vi "Validate Device ID Code.vi"(10 "Read Device ID code":T1, 11 "Device Conformity Level":T2=1 items=["None"=0, "Basic Stream"=1, "Regular Stream"=2, "Extended Stream"=3, "Basic Stream/Individual"=129, "Regular Stream/Individual"=130, "Extended Stream/Individual"=131]) -> (3 "Valid?":bool)   [LabVIEW 2014, in "MyLib.lvlib" / "Device Data Model.lvclass"]
doc: "This confirms that the device can accept the read device id request type."
uses:
  Device Data Model.lvclass
  Device ID Type.ctl
  Master Function Definition/Read Device ID code.ctl
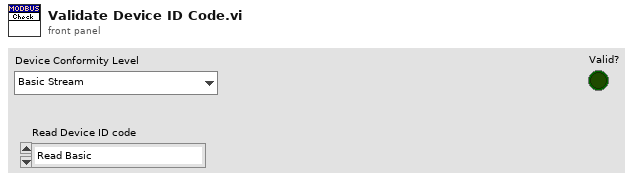
[diagram p1: front panel]
types:
  T1 = typedef "MyLib.lvlib/Device Data Model.lvclass/Read Device ID code.ctl" = enum8{"Read Basic", "Read Regular", "Read Extended", "Read Specific"}
  T2 = typedef "MyLib.lvlib/Device Data Model.lvclass/Device ID Type.ctl" = u8
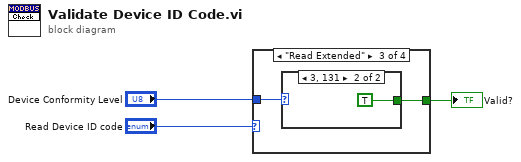
[diagram p0: block diagram]
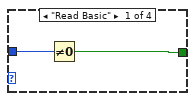
[diagram p2: hidden frame]
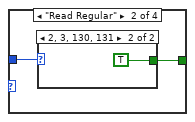
[diagram p3: hidden frame]
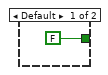
[diagram p4: hidden frame]
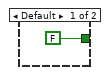
[diagram p5: hidden frame]
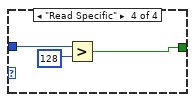
[diagram p6: hidden frame]
diagram:
  n1 = case shown="\"Read Extended\"" "Read Device ID code" {
    tunnel: "Device Conformity Level" -> [w5 w7 w11 w16]
    tunnel: [w4 w6 w10 w14] -> w1
    frame "Read Basic" {
      n2 = Not Equal To 0?(x=w5) -> (x != 0?=w4:bool)
    }
    frame "Read Regular" {
      n3 = case shown="2, 3, 130, 131" w7 {
        tunnel: [FALSE TRUE] -> w6
        frame Default {
        }
        frame 2, 3, 130, 131 {
        }
      }
    }
    frame "Read Extended" {
      n4 = case shown="3, 131" w11 {
        tunnel: [FALSE TRUE] -> w10
        frame Default {
        }
        frame 3, 131 {
        }
      }
    }
    frame "Read Specific" {
      n5 = Greater?(x=w16, y=u8 128) -> (0:w14:bool)
    }
  }
  "Valid?" <- w1
